vi "Read-all-variables.vi"(8 "error in (no error)":errorcluster, 11 "Temp. params. ref. in":refnum<data-value>) -> (0 "error out":errorcluster, 2 "Temp. vars.":T1 {"Temperature characteristics"."Stand. dev. temperature" format="%#.1f"; "Temperature characteristics"."Min. temperature" format="%#.0f"; "Temperature characteristics"."Max. temperature" format="%#.0f"; "Temperature characteristics"."Average temperature" format="%#.0f"}, 3 "Temp. params. ref.":refnum<data-value>)   [LabVIEW 2013, in "CameraVision.lvlib" / "CV-Temperature.lvclass"]
uses:
  CV-Temperature.lvclass
  Temperature-variables.ctl
  Temperature-characteristics.ctl
  UI/Module-states.ctl
  CV-Temperature.lvclass/CV-Temperature.ctl
  UI/CV-UI.lvclass
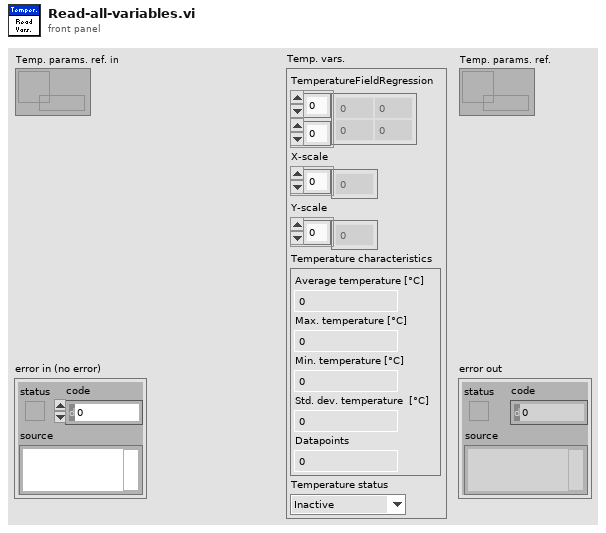
[diagram p1: front panel]
types:
  T1 = typedef "CameraVision.lvlib/CV-Temperature.lvclass/Temperature-variables.ctl" = cluster{"TemperatureFieldRegression":dbl[][], "X-scale":sgl[], "Y-scale":sgl[], "Temperature characteristics":T2, "Temperature status":T3}
  T2 = typedef "CameraVision.lvlib/CV-Temperature.lvclass/Temperature-characteristics.ctl" = cluster{"Average temperature ":dbl, "Max. temperature":dbl, "Min. temperature":dbl, "Stand. dev. temperature":dbl, "Datapoints":dbl}
  T3 = typedef "CameraVision.lvlib/CV-UI.lvclass/Module-states.ctl" = enum16{"Inactive", "Active", "Data-loss", "Error", "Simulation", "Synchronizing", "Initialized", "Released"}
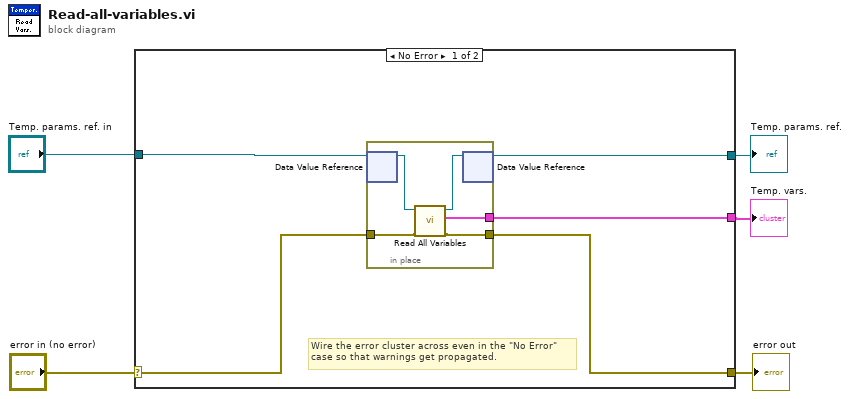
[diagram p0: block diagram]
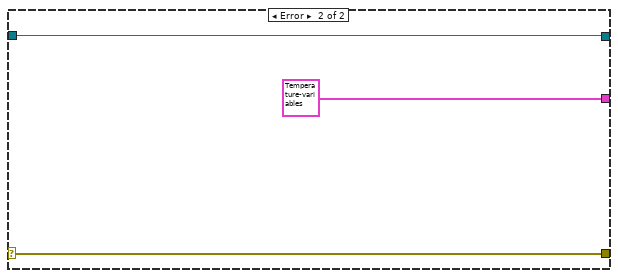
[diagram p2: hidden frame]
diagram:
  n1 = case shown="No Error" "error in (no error)" {
    selector: "error in (no error)" -> [w8 w18]
    tunnel: [w10 w18] -> w4
    tunnel: "Temp. params. ref. in" -> [w7 w16]
    tunnel: [w9 T1 {"TemperatureFieldRegression"=[], "X-scale"=[], "Y-scale"=[], "Temperature characteristics"={"Average temperature "=0.0, "Max. temperature"=0.0, "Min. temperature"=0.0, "Stand. dev. temperature"=0.0, "Datapoints"=0.0}, "Temperature status"=enum."Inactive"} ("Temp. vars.")] -> w2
    tunnel: [w6 w16] -> w1
    frame No Error {
      # "Wire the error cluster across even in the \"No Error\"\ncase so that warnings get propagated."
      n2 = in-place {
        in-place-border: [w15] -> w10
        in-place-border: [w14] -> w9
        in-place-border: w8 -> [w13]
        n3 = in-place-dvr #1(w7) -> (w12:refnum<class "CV-Temperature.lvclass">)  [unwired: 1 out]
        n4 = call "Read All Variables.vi"("error in (no error)"=w13, "Temp params in"=w12) -> ("error out"=w15:errorcluster, "Temp. vars."=w14:T1, "Temp params out"=w11:refnum<class "CV-Temperature.lvclass">)  [unwired: 7 in]
        n5 = in-place-dvr #1(w11) -> (w6:refnum<data-value>)  [unwired: 1 out]
      }
    }
    frame Error {
    }
  }
  "error out" <- w4
  "Temp. params. ref." <- w1
  "Temp. vars." <- w2
